vi "TX-ADAR-TEMP.vi"(0 "COMPORT":refnum<visa-resource-name>="COM4", 7 "RevC(t)":bool=TRUE, 11 "error in (no error)":errorcluster, 13 "Open/Close Serial":bool) -> (3 "temp 0x":string="5F", 4 "comport":refnum<visa-resource-name>="COM4", 8 "temp(c)":dbl=16.61999999999999, 15 "error out":errorcluster)   [LabVIEW 2018]
panel:
  out "cmd":string
  in  "TxPort":i32
  out "All Success":bool=TRUE
  out "output 2":string="\rwr txm 0x4A 0x70\r\n>\rrd txm 0x4B\r\n0x04B: 0x5F\r\n>"
  out "string":string="wr txm 0x4A 0x70\r\n>\nrd txm 0x4B\r\n0x04B: 0x5F\r\n>\r\n"
  out "Success":bool[](array[boolean])=[TRUE, TRUE]
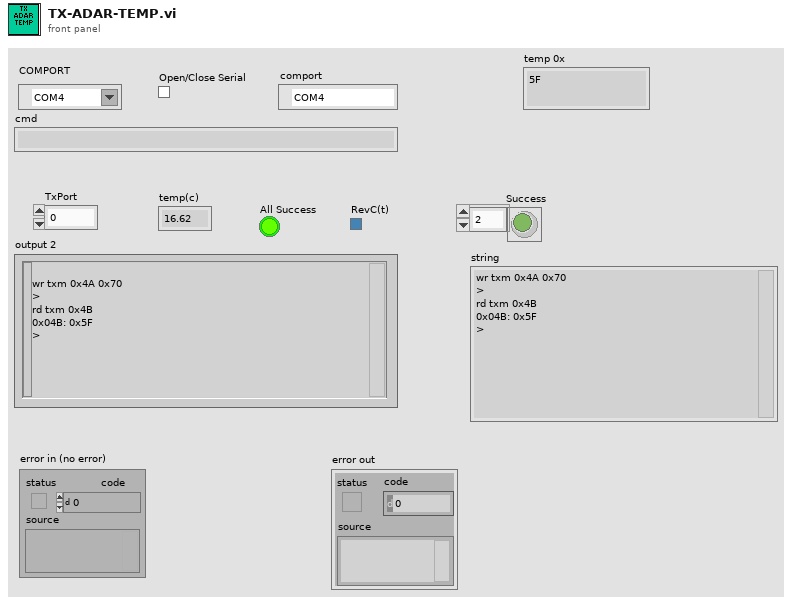
[diagram p1: front panel]
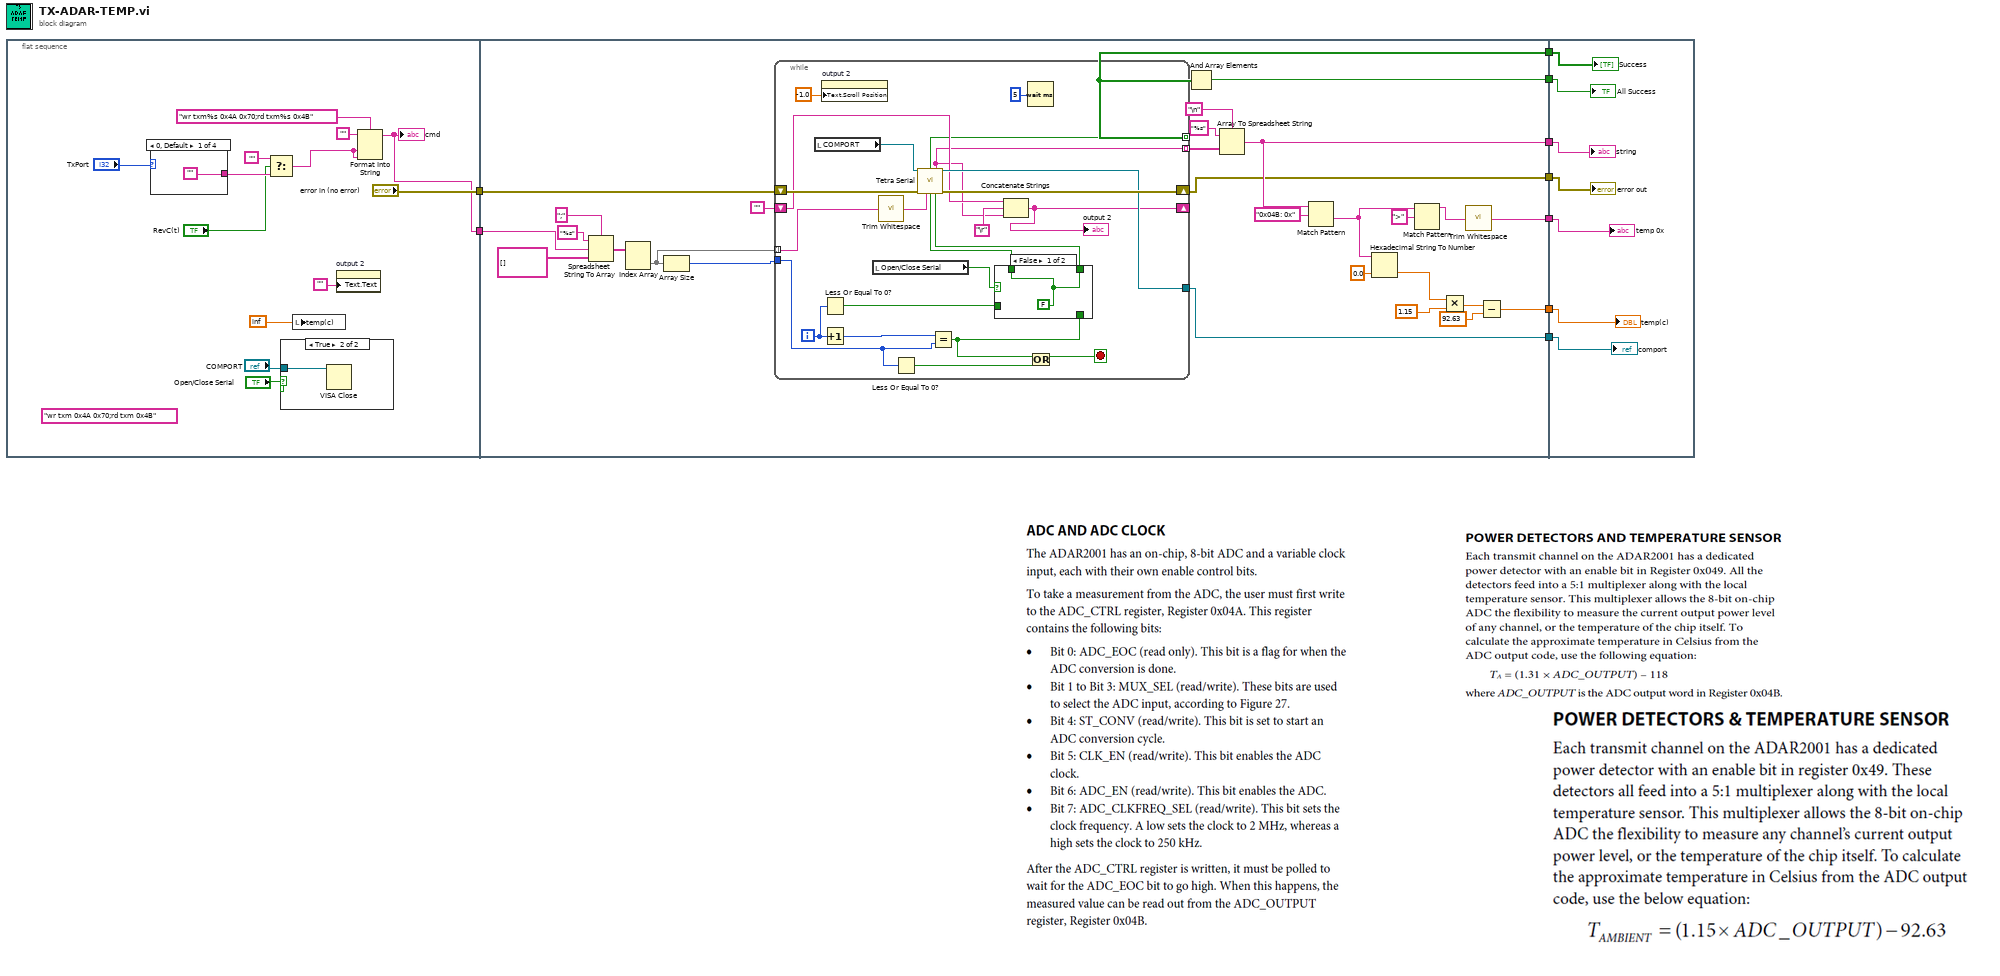
[diagram p0: block diagram]
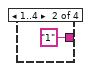
[diagram p2: hidden frame]
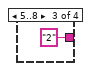
[diagram p3: hidden frame]
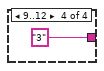
[diagram p4: hidden frame]
diagram:
  n1 = flat-sequence {
    tunnel: ["error in (no error)"] -> w9
    tunnel: [w10] -> w1
    tunnel: w9 -> [w51]
    tunnel: [w45] -> w8
    tunnel: [w44] -> w7
    tunnel: [w35] -> w6
    tunnel: [w31] -> w5
    tunnel: [w30] -> w4
    tunnel: [w29] -> w3
    tunnel: [w28] -> w2
    tunnel: w1 -> [w47]
    tunnel: w8 -> [w82]
    tunnel: w7 -> [w83]
    tunnel: w6 -> [w85]
    tunnel: w5 -> [w84]
    tunnel: w4 -> [w86]
    tunnel: w3 -> [w87]
    tunnel: w2 -> [w88]
    frame #0 {
      (unwired) "wr txm 0x4A 0x70;rd txm 0x4B" ("Command ( ; seperation)")
      n2 = case shown="0, Default" "TxPort" {
        tunnel: ["" "1" "2" "3"] -> w14
        frame 0, Default {
        }
        frame 1..4 {
        }
        frame 5..8 {
        }
        frame 9..12 {
        }
      }
      n3 = Select(t="", s="RevC(t)", f=w14) -> (s? t:f=w13:string)
      n4 = case shown="True" "Open/Close Serial" {
        tunnel: "COMPORT" -> [_ w27]
        frame False {
        }
        frame True {
          n5 = VISA Close(VISA resource name=w27) -> ()  [unwired: 1 in, 1 out]
        }
      }
      n6 = local write "temp(c)"(inf) -> ()
      n7 = property on="output 2" class="Str"("Text.Text"="") -> ()  [unwired: 2 in, 2 out]
      n8 = Format Into String(format string="wr txm%s 0x4A 0x70;rd txm%s 0x4B" ("Command ( ; seperation)"), initial string="", w13, w13) -> (resulting string=w10:string)  [unwired: 1 in, 1 out]
      "cmd" <- w10
    }
    frame #1 {
      n9 = Spreadsheet String To Array(delimiter (Tab)=";", format string="%s", spreadsheet string=w47, array type (2D Dbl)=string[][] []) -> (array=w52:string[][])
      n10 = Index Array(array=w52) -> (element=w50:string[])  [unwired: 2 in]
      n11 = Array Size(array=w50) -> (size(s)=w42:i32)
      n12 = while {
        shift-right: [w78] -> w28
        shift-left: w51 -> [w77]
        tunnel: [w71] -> w43 mode=indexing
        tunnel: w50 -> [w75] mode=indexing
        tunnel: w42 -> [w64]
        shift-right: [w68] -> _
        shift-left: "" -> [w72]
        tunnel: [w69] -> w45 mode=indexing
        tunnel: [w76] -> w30
        i -> [w66]
        stop <- w65 stop-if-true
        n13 = local read "COMPORT"() -> (w56:refnum<visa-resource-name>)
        n14 = property on="output 2" class="Str"("Text.Scroll Position"=-1.0) -> ()  [unwired: 2 in, 2 out]
        n15 = Less Or Equal To 0?(x=w66) -> (x <= 0?=w60:bool)
        n16 = Increment(x=w66) -> (x+1=w67:i32)
        n17 = local read "Open/Close Serial"() -> (w57:bool)
        n18 = call <vilib>:"Trim Whitespace.vi"("string"=w75) -> ("trimmed string"=w70:string)  [unwired: 1 in]
        n19 = Less Or Equal To 0?(x=w64) -> (x <= 0?=w63:bool)
        n20 = Equal?(x=w67, y=w64) -> (x = y?=w58:bool)
        n21 = case shown="False" w57 {
          tunnel: [w79 w81] -> w61
          tunnel: w60 -> [_ w81]
          tunnel: [w79 w80] -> w59
          tunnel: w58 -> [_ w80]
          frame False {
            w79 = FALSE
          }
          frame True {
          }
        }
        n22 = call "Tetra Serial.vi"("COMPORT"=w56, "error in (no error)"=w77, "Command"=w70, "Open Ser(t)"=w61, "Close Ser(t)"=w59) -> ("Success"=w69:bool, "output"=w71:string, "comport"=w76:refnum<visa-resource-name>, "error out"=w78:errorcluster)  [unwired: 6 in, 1 out]
        n23 = Concatenate Strings(w72, "\r", w71) -> (w68:string)
        "output 2" <- w68
        n24 = Wait (ms)(milliseconds to wait=u32 5) -> ()  [unwired: 1 out]
        n25 = Or(x=w58, y=w63) -> (x .or. y?=w65:bool)
      }
      n26 = And Array Elements(Boolean array=w45) -> (logical AND=w44:bool)
      n27 = Array To Spreadsheet String(delimiter (Tab)="\n", array=w43, 3:"%s" ("format string")) -> (spreadsheet string=w29:string)
      n28 = Match Pattern(string=w29, regular expression="0x04B: 0x") -> (after substring=w34:string)  [unwired: 1 in, 3 out]
      n29 = Hexadecimal String To Number(string=w34, default (0uL)=0.0 ("default (0 U32)")) -> (number=w39:dbl)  [unwired: 1 in, 1 out]
      n30 = Match Pattern(string=w34, regular expression=">") -> (before substring=w32:string)  [unwired: 1 in, 3 out]
      n31 = Multiply(x=w39, y=1.15) -> (x*y=w37:dbl)
      n32 = call <vilib>:"Trim Whitespace.vi"("string"=w32) -> ("trimmed string"=w31:string)  [unwired: 1 in]
      n33 = Subtract(x=w37, y=92.63) -> (x-y=w35:dbl)
    }
    frame #2 {
      "Success" <- w82
      "All Success" <- w83
      "temp 0x" <- w84
      "temp(c)" <- w85
      "comport" <- w86
      "string" <- w87
      "error out" <- w88
    }
  }
